vi "Main_simpler_algorithm.vi"() -> ()   [LabVIEW 2018]
uses:
  <vilib>/Analysis/NI_AALBase.lvlib
panel:
  out "EtuliikeKielletty?":bool
  out "90asteenkäännös":bool
  in  "Count Integer 2":i32
  out "MedianPingOikea":dbl format="%0.2f"
  out "OikeaPing(cm)":dbl
  in  "Count Integer":i32
  out "MedianPingVasen":dbl format="%0.2f"
  out "VasenPing(cm)":dbl
  out "Käännökset":dbl
  out "Takadist":dbl
  out "EtuDist":dbl
  out "TakaSpeedTaakse":dbl
  out "EtuSpeedTaakse":dbl
  out "OikeaSpeedTaakse":dbl
  out "VasenSpeedTaakse":dbl
  out "OikeaDist":dbl
  out "VasenDist":dbl
  out "VasenSpeedEteen":dbl
  out "OikeaSpeedEteen":dbl
  out "TakaSpeedEteen":dbl
  out "EtuSpeedEteen":dbl
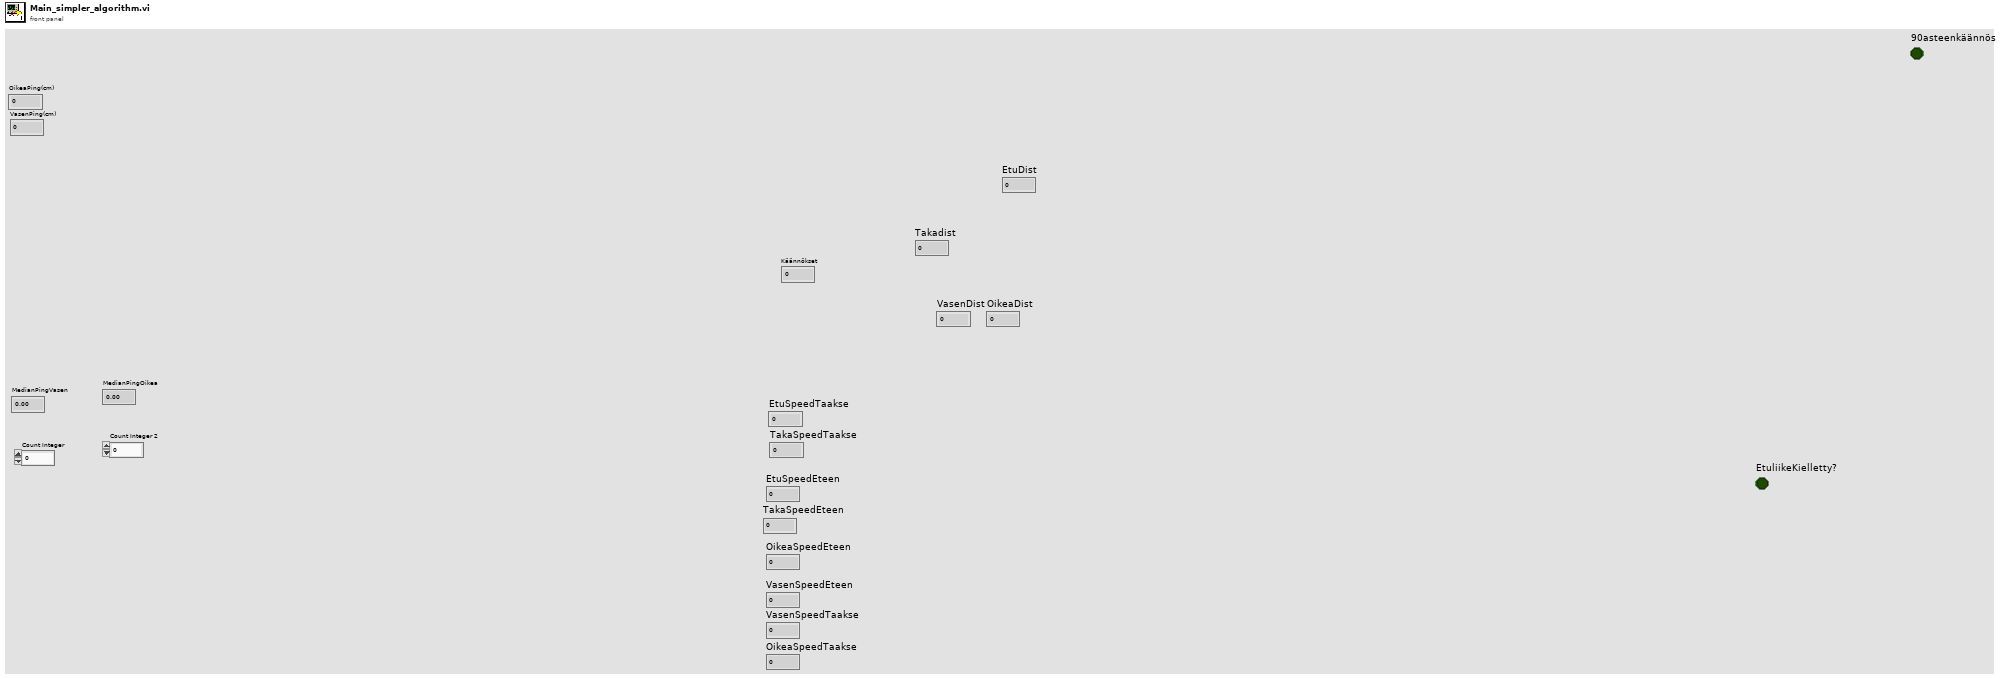
[diagram p1: front panel]
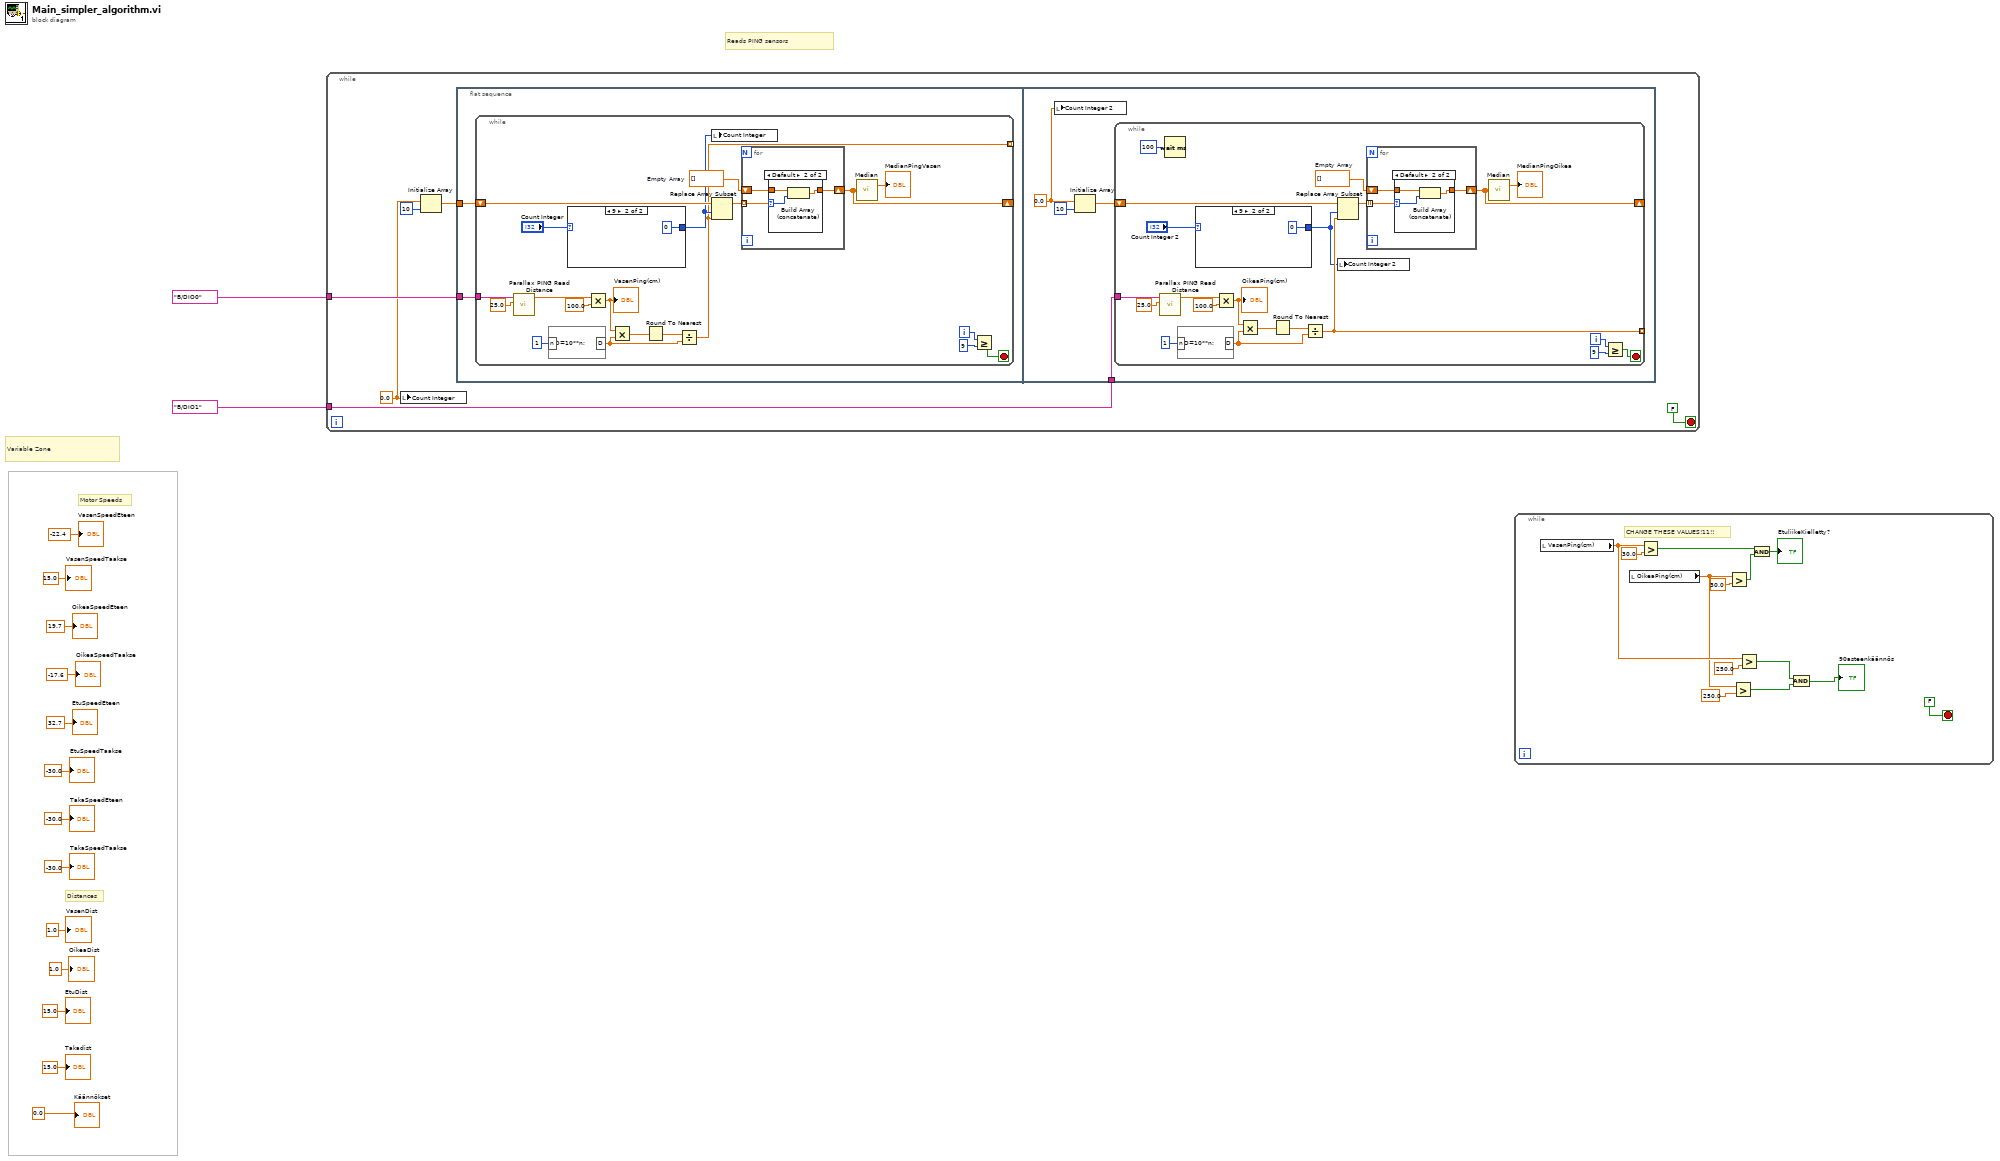
[diagram p0: block diagram]
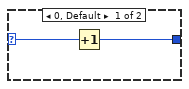
[diagram p3: hidden frame]
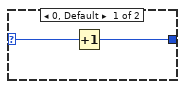
[diagram p5: hidden frame]
diagram:
  # "Reads PING sensors"
  # "Variable Zone"
  # "Motor Speeds"
  # "Distances"
  n1 = while {
    tunnel: tag "B/DIO0" ("myRIO DIO Channel") -> [w21]
    tunnel: tag "B/DIO1" ("myRIO DIO Channel") -> [w20]
    stop <- FALSE stop-if-true
    w18 = 0.0 ("element")
    n2 = local write "Count Integer"(w18) -> ()
    n3 = Initialize Array(w18, 10 ("dimension size")) -> (w16:dbl[])
    n4 = flat-sequence {
      tunnel: w16 -> [w23]
      tunnel: w21 -> [w22]
      tunnel: w20 -> [w57]
      frame #0 {
        n5 = while {
          shift-right: [w25] -> _
          shift-left: w23 -> [w43]
          tunnel: [w36] -> _ mode=indexing
          tunnel: w22 -> [w32]
          i -> [w29]
          stop <- w30 stop-if-true
          w27 = dbl[] []  # Empty Array
          n6 = call "Parallax PING Read Distance.vi"("Temperature (deg C)"=25.0, "myRIO DIO Channel"=w32) -> ("Distance (m)"=w34:dbl)  [unwired: 8 in, 1 out]
          n7 = formula code="D=10**n;"("n"=u16 1 ("input variable")) -> ("D"=w38:dbl)
          n8 = case shown="9" "Count Integer" {
            selector: "Count Integer" -> [w52 _]
            tunnel: [w51 0] -> w41
            frame 0, Default {
              n9 = Increment(x=w52) -> (x+1=w51:i32)
            }
            frame 9 {
            }
          }
          n10 = Multiply(x=w34, y=100.0 ("Temperature (deg C)")) -> (x*y=w28:dbl)
          "VasenPing(cm)" <- w28
          n11 = Multiply(x=w28, y=w38) -> (x*y=w40:dbl)
          n12 = Round To Nearest(number=w40) -> (nearest integer value=w39:dbl)
          n13 = Divide(x=w39, y=w38) -> (x/y=w36:dbl)
          n14 = local write "Count Integer"(w41) -> ()
          n15 = Replace Array Subset(array=w43, new element=w36, index=w41) -> (w26:dbl[])
          n16 = for {
            shift-right: [w45] -> w25
            shift-left: w27 -> [w46]
            tunnel: w26 -> [w44] mode=indexing
            n17 = case shown="Default" w44 {
              selector: w44 -> [_ w48]
              tunnel: w46 -> [w47 w50]
              tunnel: [w47 w49] -> w45
              frame 0 {
              }
              frame Default {
                n18 = Build Array (concatenate)(w50, w48) -> (w49:dbl[])
              }
            }
          }
          n19 = call <vilib>:"Median.vi"("X"=w25) -> ("median"=→"MedianPingVasen":dbl)  [unwired: 1 out]
          n20 = Greater Or Equal?(x=w29, y=9) -> (x >= y?=w30:bool)
        }
      }
      frame #1 {
        w55 = 0.0 ("element")
        n21 = local write "Count Integer 2"(w55) -> ()
        n22 = Initialize Array(w55, 10 ("dimension size")) -> (w54:dbl[])
        n23 = while {
          shift-right: [w59] -> _
          shift-left: w54 -> [w78]
          tunnel: [w71] -> _ mode=indexing
          tunnel: w57 -> [w67]
          i -> [w65]
          stop <- w66 stop-if-true
          w61 = dbl[] []  # Empty Array
          n24 = call "Parallax PING Read Distance.vi"("Temperature (deg C)"=25.0, "myRIO DIO Channel"=w67) -> ("Distance (m)"=w69:dbl)  [unwired: 8 in, 1 out]
          n25 = Wait (ms)(milliseconds to wait=u32 100) -> ()  [unwired: 1 out]
          n26 = formula code="D=10**n;"("n"=u16 1 ("input variable")) -> ("D"=w73:dbl)
          n27 = case shown="9" "Count Integer 2" {
            selector: "Count Integer 2" -> [w87 _]
            tunnel: [w86 0] -> w63
            frame 0, Default {
              n28 = Increment(x=w87) -> (x+1=w86:i32)
            }
            frame 9 {
            }
          }
          n29 = Multiply(x=w69, y=100.0 ("Temperature (deg C)")) -> (x*y=w62:dbl)
          "OikeaPing(cm)" <- w62
          n30 = Multiply(x=w62, y=w73) -> (x*y=w75:dbl)
          n31 = Round To Nearest(number=w75) -> (nearest integer value=w74:dbl)
          n32 = Divide(x=w74, y=w73) -> (x/y=w71:dbl)
          n33 = Replace Array Subset(array=w78, new element=w71, index=w63) -> (w60:dbl[])
          n34 = local write "Count Integer 2"(w63) -> ()
          n35 = for {
            shift-right: [w79] -> w59
            shift-left: w61 -> [w80]
            tunnel: w60 -> [w81] mode=indexing
            n36 = case shown="Default" w81 {
              selector: w81 -> [_ w83]
              tunnel: w80 -> [w82 w85]
              tunnel: [w82 w84] -> w79
              frame 0 {
              }
              frame Default {
                n37 = Build Array (concatenate)(w85, w83) -> (w84:dbl[])
              }
            }
          }
          n38 = call <vilib>:"Median.vi"("X"=w59) -> ("median"=→"MedianPingOikea":dbl)  [unwired: 1 out]
          n39 = Greater Or Equal?(x=w65, y=9) -> (x >= y?=w66:bool)
        }
      }
    }
  }
  n40 = while {
    stop <- FALSE stop-if-true
    # "CHANGE THESE VALUES!11!!"
    n41 = local read "VasenPing(cm)"() -> (w96:dbl)
    n42 = local read "OikeaPing(cm)"() -> (w95:dbl)
    n43 = Greater?(x=w96, y=30.0 ("t")) -> (0:w99:bool)
    n44 = Greater?(x=w95, y=30.0 ("t")) -> (0:w100:bool)
    n45 = Greater?(x=w95, y=250.0 ("t")) -> (0:w90:bool)
    n46 = Greater?(x=w96, y=250.0 ("t")) -> (0:w91:bool)
    n47 = And(x=w99, y=w100) -> (x .and. y?=→"EtuliikeKielletty?":bool)
    n48 = And(x=w91, y=w90) -> (x .and. y?=→"90asteenkäännös":bool)
  }
  "EtuSpeedEteen" <- 32.7 ("t")
  "TakaSpeedEteen" <- -30.0 ("t")
  "OikeaSpeedEteen" <- 19.7 ("t")
  "VasenSpeedEteen" <- -22.4 ("t")
  "VasenDist" <- 1.0 ("VasenDist")
  "OikeaDist" <- 1.0 ("VasenDist")
  "VasenSpeedTaakse" <- 15.0 ("t")
  "OikeaSpeedTaakse" <- -17.6 ("t")
  "EtuSpeedTaakse" <- -30.0 ("t")
  "TakaSpeedTaakse" <- -30.0 ("t")
  "EtuDist" <- 15.0 ("EtuDist")
  "Takadist" <- 15.0 ("EtuDist")
  "Käännökset" <- 0.0 ("Käännökset")
